vi "Logger.vi"(7 "Plugin Name":string, 8 "error in":errorcluster, 9 "Log":T1={"Message"="", "Level"=enum."Error", "Add to log file? (F)"=FALSE, "Append newline? (T)"=TRUE}, 10 "State":enum16{"Initialize", "Log"}(ring), 11 "Template in":refnum<class "Template.lvclass">) -> (0 "error out":errorcluster, 3 "Template out":refnum<class "Template.lvclass">)   [LabVIEW 2026, in "Template Plugin.lvlib" / "Template.lvclass"]
uses:
  Template.lvclass
  Template.lvclass/Template.ctl
  <userlib>/CustomDeviceInterfaces_v1.lvlibp/custom-device-express-framework/Source/Custom Device Interfaces/CustomDeviceAPI/CustomDeviceAPI.lvclass
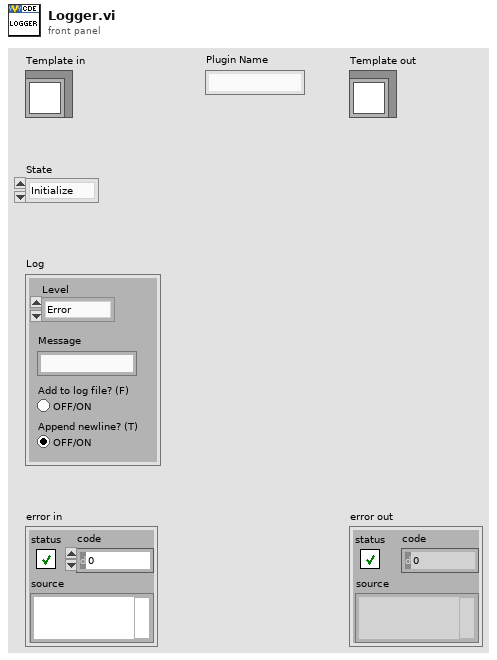
[diagram p1: front panel]
types:
  T1 = cluster{"Message":string, "Level":enum16{"Error", "Warning", "Info", "Debug"}, "Add to log file? (F)":bool, "Append newline? (T)":bool}
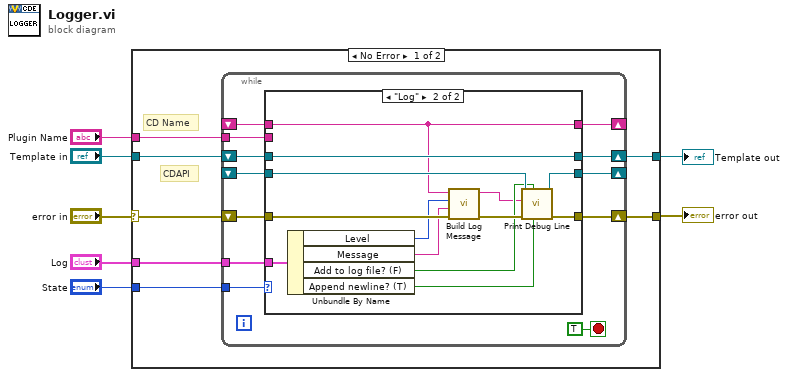
[diagram p0: block diagram]
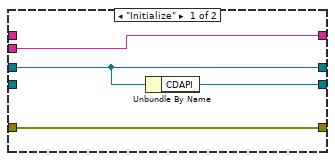
[diagram p2: hidden frame]
diagram:
  n1 = case shown="No Error" "error in" {
    selector: "error in" -> [w14 w45]
    tunnel: "Template in" -> [w12 w44]
    tunnel: [w11 w44] -> w4
    tunnel: "State" -> [w10 _]
    tunnel: [w13 w45] -> w6
    tunnel: "Log" -> [w9 _]
    tunnel: "Plugin Name" -> [w8 _]
    frame No Error {
      # "CDAPI"
      # "CD Name"
      n2 = while {
        shift-right: [w23] -> w11
        shift-left: w12 -> [w20]
        tunnel: w10 -> [w24]
        shift-right: [w22] -> _
        shift-left: _ -> [w21]
        shift-right: [w25] -> w13
        shift-left: w14 -> [w26]
        tunnel: w9 -> [w19]
        tunnel: w8 -> [w18]
        shift-right: [w17] -> _
        shift-left: _ -> [w16]
        stop <- TRUE stop-if-true
        n3 = case shown="\"Log\"" w24 {
          tunnel: w20 -> [w28 w40]
          tunnel: [w28 w40] -> w23
          tunnel: [w29 w31] -> w22
          tunnel: w21 -> [_ w39]
          tunnel: w26 -> [w30 w42]
          tunnel: [w30 w43] -> w25
          tunnel: w19 -> [_ w38]
          tunnel: w18 -> [w27 _]
          tunnel: [w27 w32] -> w17
          tunnel: w16 -> [_ w32]
          frame "Initialize" {
            n4 = Unbundle By Name(w28) -> ("CDAPI"=w29:refnum<class "CustomDeviceAPI.lvclass">)
          }
          frame "Log" {
            n5 = Unbundle By Name(w38) -> ("Level"=w34:enum16{"Error", "Warning", "Info", "Debug"}, "Message"=w33:string, "Add to log file? (F)"=w37:bool, "Append newline? (T)"=w36:bool)
            n6 = call "Build Log Message.vi"("error in"=w42, "Message"=w33, "Level"=w34, "Plugin Name"=w32) -> ("error out"=w41:errorcluster, "Log Message"=w35:string)  [unwired: 6 in]
            n7 = call-dynamic "Print Debug Line.vi"("Append newline? (T)"=w36, "Add to log file? (F)"=w37, "error in"=w41, "Message"=w35, "iCDAPI in"=w39) -> ("error out"=w43:errorcluster, "iCDAPI out"=w31:refnum<class "CustomDeviceAPI.lvclass">)  [unwired: 5 in]
          }
        }
      }
    }
    frame Error {
    }
  }
  "Template out" <- w4
  "error out" <- w6
